vi "Encoder Position Estimate.vi"(9 "Last Vision Y":dbl, 11 "Last Vision X":dbl) -> (1 "Y":dbl, 3 "X":dbl)   [LabVIEW 2013]
uses:
  <vilib>/Analysis/coordinate.llb/2D Cartesian Coordinate Rotation (Scalar).vi
  Common Code/Change Detect Boolean.vi
  Robot Global Data.vi
  <vilib>/Rock Robotics/WPI/Gyro/WPI_GyroRefNum Registry Get.vi
  <vilib>/Rock Robotics/WPI/Gyro/WPI_GyroGetAngle.vi
  <vilib>/Analysis/NI_AALPro.lvlib
panel:
  in  "Estimate Pos":bool
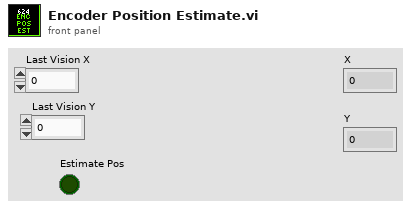
[diagram p1: front panel]
types:
  T1 = typedef "Encoder Data.ctl" = cluster{"Avg Distance L/R":dbl, "Avg Speed L/R":dbl, "Left":T2, "Right":T2, "Omni":T2}
  T2 = typedef "Single Encoder Data.ctl" = cluster{"Distance":dbl, "Speed":dbl, "Ticks":dbl}
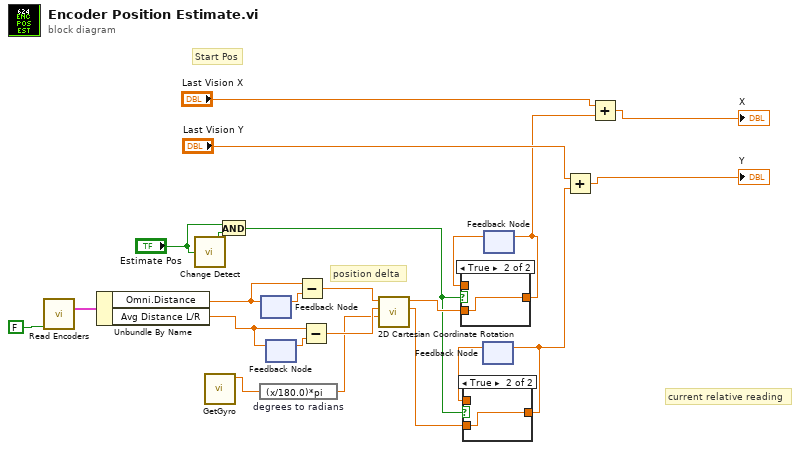
[diagram p0: block diagram]
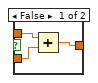
[diagram p2: hidden frame]
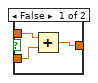
[diagram p3: hidden frame]
diagram:
  # "position delta"
  # "current relative reading"
  # "Start Pos"
  n1 = call "Read Encoders.vi"("Reset"=FALSE) -> ("Encoder Data"=w22:T1)  [unwired: 10 in]
  n2 = Unbundle By Name(w22) -> ("Omni.Distance"=w15:dbl, "Avg Distance L/R"=w13:dbl)
  n3 = call-poly "Change Detect.vi"("In"="Estimate Pos") -> ("Changed?"=w17:bool)
  n4 = call "GetGyro.vi"() -> ("Angle"=w9:dbl)  [unwired: 10 in, 1 out]
  n5 = And(x="Estimate Pos", y=w17) -> (x .and. y?=w3:bool)
  n6 = expression code="(x/180.0)*pi" "degrees to radians"(w9) -> (w8:dbl)
  n7 = feedback-in #1(w15) -> ()
  n8 = feedback #1() -> (w14:dbl)  [unwired: 1 in]
  n9 = feedback #2() -> (w12:dbl)  [unwired: 1 in]
  n10 = feedback-in #2(w13) -> ()
  n11 = Subtract(x=w15, y=w14) -> (x-y=w11:dbl)
  n12 = Subtract(x=w13, y=w12) -> (x-y=w10:dbl)
  n13 = call-poly <vilib>:"2D Cartesian Coordinate Rotation.vi"("theta"=w8, "y"=w10, "x"=w11) -> ("y out"=w5:dbl, "x out"=w7:dbl)  [unwired: 6 in, 1 out]
  n14 = feedback #3() -> (w4:dbl)  [unwired: 1 in]
  n15 = case shown="True" w3 {
    tunnel: w5 -> [w26 w27]
    tunnel: [w24 w27] -> w1
    tunnel: w4 -> [w25 _]
    frame False {
      n16 = Add(x=w25, y=w26) -> (x+y=w24:dbl)
    }
    frame True {
    }
  }
  n17 = feedback-in #3(w1) -> ()
  n18 = feedback #4() -> (w6:dbl)  [unwired: 1 in]
  n19 = case shown="True" w3 {
    tunnel: w7 -> [w30 w31]
    tunnel: [w28 w31] -> w2
    tunnel: w6 -> [w29 _]
    frame False {
      n20 = Add(x=w29, y=w30) -> (x+y=w28:dbl)
    }
    frame True {
    }
  }
  n21 = feedback-in #4(w2) -> ()
  n22 = Add(x="Last Vision Y", y=w1) -> (x+y=→"Y":dbl)
  n23 = Add(x="Last Vision X", y=w2) -> (x+y=→"X":dbl)
